vi "Vision_linedetection.vi"   [LabVIEW 2019]
uses:
  Global Var.vi
types:
  T1 = typedef "IMAQ Image.ctl" = refnum<image>
  T2 = cluster{"Point1 (Pixels)":cluster{"X":sgl, "Y":sgl}, "Point2 (Pixels)":cluster{"X":sgl, "Y":sgl}, "Point1 (Real-World)":cluster{"X":sgl, "Y":sgl}, "Point2 (Real-World)":cluster{"X":sgl, "Y":sgl}, "Angle (Pixel)":dbl, "Angle (Real-World)":dbl, "Score":dbl, "Straightness":dbl, "Average SNR (db)":dbl, "Calibration Valid":bool}
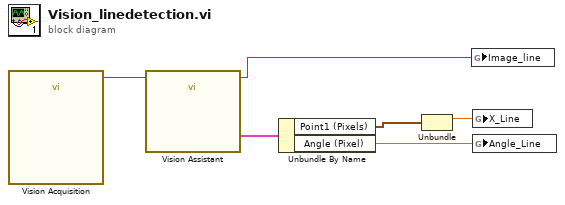
[diagram p0: block diagram]
diagram:
  n1 = call "Vision Acquisition"() -> ("Image Out"=w2:T1)  [unwired: 25 in, 2 out]
  n2 = call "Vision Assistant"("Image In"=w2) -> ("Image Out"=w1:T1, "Straight Edge (Find Straight Edge 1)"=w6:T2)  [unwired: 24 in, 1 out]
  n3 = Unbundle By Name(w6) -> ("Point1 (Pixels)"=w5:cluster{"X":sgl, "Y":sgl}, "Angle (Pixel)"=w3:dbl)
  n4 = Unbundle(w5) -> ("X"=w4:sgl)  [unwired: 1 out]
  n5 = global write "Global Var.vi" "Image_line"(w1) -> ()
  n6 = global write "Global Var.vi" "X_Line"(w4) -> ()
  n7 = global write "Global Var.vi" "Angle_Line"(w3) -> ()
